vi "Wait for MS Motor.vi"(0 "Timeout":dbl, 5 "Wait For On/Off?":bool, 11 "Error In":errorcluster) -> (4 "Pass/Fail?":bool, 6 "Report Text":string, 15 "Error Out":errorcluster)   [LabVIEW 2016, in "2015 VA Washer.lvlib"]
uses:
  Projects/2015 VA Washer.lvlib
  <vilib>/DAQmx/read.llb/DAQmx Read (Digital Bool 1Line 1Point).vi
  <vilib>/DAQmx/create/channels.llb/DAQmx Create Channel (DI-Digital Input).vi
  <vilib>/DAQmx/miscellaneous.llb/DAQmx Fill In Error Info.vi
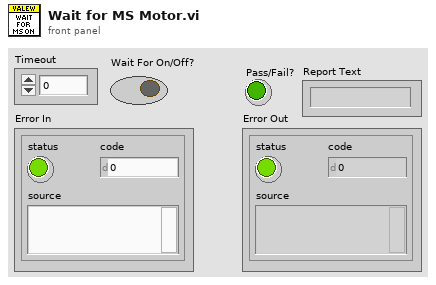
[diagram p1: front panel]
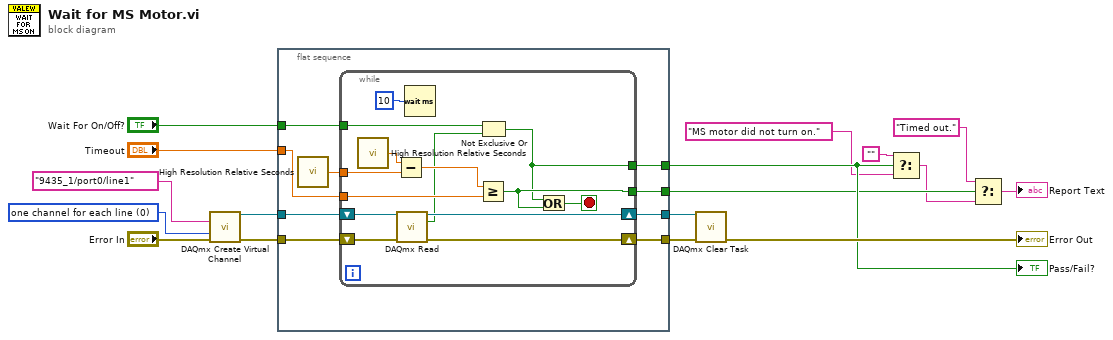
[diagram p0: block diagram]
diagram:
  w15 = 0 items=["one channel for each line", "one channel for all lines"] ("line grouping")
  n1 = call-poly <vilib>:"DAQmx Create Virtual Channel.vi"("lines"=tag "9435_1/port0/line1", "line grouping"=w15, "error in"="Error In") -> ("task out"=w17:refnum<k21>, "error out"=w14:errorcluster)  [unwired: 11 in]
  n2 = flat-sequence {
    tunnel: w17 -> [w26]
    tunnel: w14 -> [w25]
    tunnel: [w23] -> w12
    tunnel: [w22] -> w11
    tunnel: [w21] -> w8
    tunnel: "Timeout" -> [w20]
    tunnel: [w19] -> w5
    tunnel: "Wait For On/Off?" -> [w18]
    frame #0 {
      n3 = call <vilib>:"High Resolution Relative Seconds.vi"() -> ("relative seconds"=w24:dbl)
      n4 = while {
        shift-right: [w37] -> w23
        shift-left: w26 -> [w40]
        shift-right: [w38] -> w22
        shift-left: w25 -> [w39]
        tunnel: w24 -> [w35]
        tunnel: [w27] -> w21
        tunnel: w20 -> [w31]
        tunnel: [w30] -> w19
        tunnel: w18 -> [w29]
        stop <- w33 stop-if-true
        n5 = call <vilib>:"High Resolution Relative Seconds.vi"() -> ("relative seconds"=w36:dbl)
        n6 = Subtract(x=w36, y=w35) -> (x-y=w34:dbl)
        n7 = call-poly <vilib>:"DAQmx Read.vi"("task/channels in"=w40, "error in"=w39) -> ("task out"=w37:refnum<k21>, "data"=w28:bool, "error out"=w38:errorcluster)  [unwired: 11 in]
        n8 = Wait (ms)(milliseconds to wait=u32 10) -> ()  [unwired: 1 out]
        n9 = Greater Or Equal?(x=w34, y=w31) -> (x >= y?=w30:bool)
        n10 = Not Exclusive Or(1:w28, 2:w29) -> (0:w27:bool)
        n11 = Or(x=w27, y=w30) -> (x .or. y?=w33:bool)
      }
    }
  }
  n12 = call <vilib>:"DAQmx Clear Task.vi"("task in"=w12, "error in"=w11) -> ("error out"=→"Error Out":errorcluster)  [unwired: 13 in]
  n13 = Select(t="", s=w8, f="MS motor did not turn on.") -> (s? t:f=w4:string)
  n14 = Select(t="Timed out." ("f"), s=w5, f=w4) -> (s? t:f=→"Report Text":string)
  "Pass/Fail?" <- w8
